vi "QCA - DUT Generate Tx Command Dll.vi"(10 "TestItem_Index":i32, 11 "File Path String":string) -> (0 "ChainSet_ch":i32, 1 "FreqSet_f":i32, 2 "RateSet_r":i32[](array[numeric]), 3 "Command Sent":string, 4 "Standard_Index":i32)   [LabVIEW 2011]
panel:
  out "Total Test Items":i32
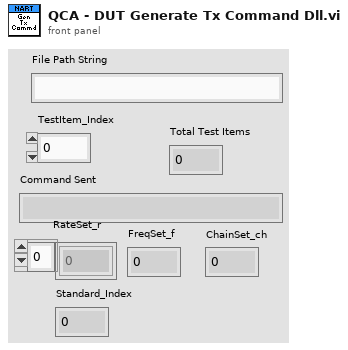
[diagram p1: front panel]
types:
  T1 = typedef "WLAN - TV - RW - INC - TV_DataType_Cluster.ctl" = cluster{"Standard":i32, "Channel Frequency(Hz)":dbl, "Power Level(dBm)":dbl, "Channel Bandwidth (Hz)":dbl, "Idle Interval(s)":dbl, "OFDM Data Rate (Mbps)":i32, "OFDM Payload Length (bytes)":i32, "Number of Packets":i32, "MCS Index":i32, "Guard Interval (s)":dbl, "80211n PLCP Frame Format":i32, "FEC Coding Type":i32, "DSSS Data Rate (Mbps)":i32, "DSSS Payload Length (bytes)":i32, "N_SS":i32, "Tx_Chan":u32}
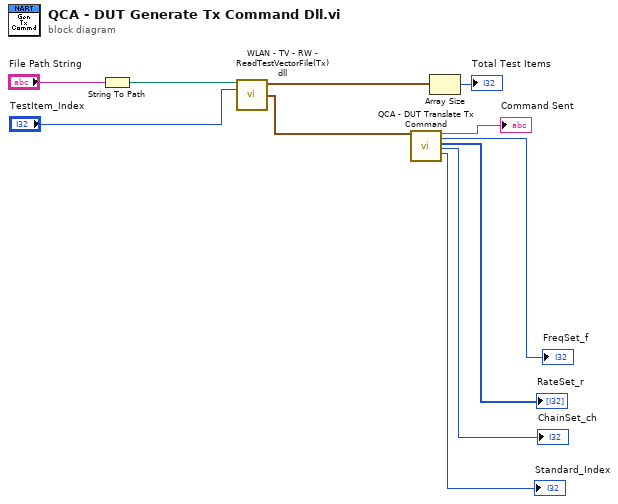
[diagram p0: block diagram]
diagram:
  n1 = String To Path(string="File Path String") -> (path=w8:path)
  n2 = call "WLAN - TV - RW - ReadTestVectorFile(Tx) dll.vi"("file path (dialog if empty)"=w8, "TestItem_Index"="TestItem_Index") -> ("TV's"=w10:T1[], "Current TV Element"=w6:T1)  [unwired: 11 in, 1 out]
  n3 = call "QCA - DUT Translate Tx Command.vi"("TV Parameters(DataType)"=w6) -> ("Command Sent"=→"Command Sent":string, "FreqSet_f"=→"FreqSet_f":i32, "RateSet_r"=→"RateSet_r":i32[], "ChainSet_ch"=→"ChainSet_ch":i32, "Standard_Index"=→"Standard_Index":i32)  [unwired: 13 in, 1 out]
  n4 = Array Size(array=w10) -> (size(s)=→"Total Test Items":i32)
